vi "mydaq_equalizer.vi"() -> ()   [LabVIEW 2018]
uses:
  <vilib>/express/express analysis/Spectral/Block/exnSpectralBlock spectral measurements power poly.vi
  <vilib>/express/express analysis/Spectral/Block/exnSpectralBlock spectral measurements power DDT.vi
  <vilib>/express/express analysis/Spectral/XNode/ExpressSpectralMeasurementsBlockNode.xnode
panel:
  out "Waveform Graph":dynamicdata(graph)
  in  "Volume":dbl(slide) scale=0.0..1.0
  out "Slide 3":dbl(slide) scale=0.002..2.0
  out "Slide 2":dbl(slide) scale=0.002..2.0
  out "Slide":dbl(slide) scale=0.008..8.0
  in  "Bass":dbl(slide) scale=0.0..1.0
  in  "Midtone":dbl(slide) scale=0.0..1.0
  in  "Treble":dbl(slide)=0.5 scale=0.0..1.0
  in  "stop (F)":bool
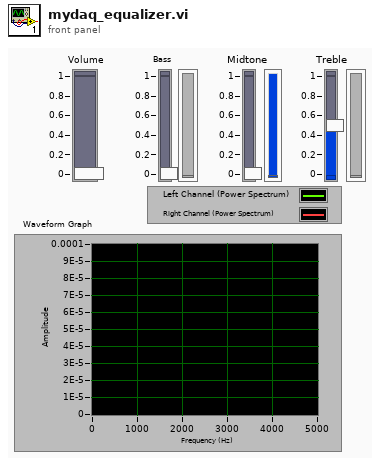
[diagram p1: front panel]
types:
  T1 = cluster{"averaging mode":u16, "weighting mode":u16, "number of averages":u32}
  T2 = cluster{"dB On (F)":bool, "unwrap phase (F)":bool, "convert to degree (F)":bool}
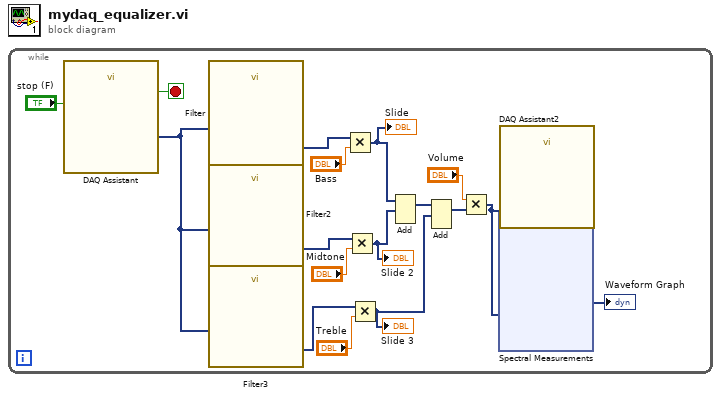
[diagram p0: block diagram]
diagram:
  n1 = while {
    stop <- w17 stop-if-true
    n2 = call "DAQ Assistant"("stop (F)"="stop (F)") -> ("data"=w15:dynamicdata, "stopped"=w17:bool)  [unwired: 15 in, 2 out]
    n3 = call "Filter"("Signal"=w15) -> ("Filtered Signal"=w11:dynamicdata)  [unwired: 9 in, 1 out]
    n4 = call "Filter2"("Signal"=w15) -> ("Filtered Signal"=w13:dynamicdata)  [unwired: 9 in, 1 out]
    n5 = call "Filter3"("Signal"=w15) -> ("Filtered Signal"=w9:dynamicdata)  [unwired: 9 in, 1 out]
    n6 = Multiply(x=w11, y="Bass") -> (x*y=w6:dynamicdata)
    "Slide" <- w6
    n7 = Multiply(x=w13, y="Midtone") -> (x*y=w5:dynamicdata)
    "Slide 2" <- w5
    n8 = Multiply(x=w9, y="Treble") -> (x*y=w7:dynamicdata)
    "Slide 3" <- w7
    n9 = Add(1:w5, 2:w6) -> (0:w14:dynamicdata)  [unwired: 1 in, 1 out]
    n10 = Add(1:w7, 2:w14) -> (0:w2:dynamicdata)  [unwired: 1 in, 1 out]
    n11 = Multiply(x="Volume", y=w2) -> (x*y=w4:dynamicdata)
    n12 = xnode "Spectral Measurements"("Signals"=w4) -> ("Power Spectrum"=→"Waveform Graph":dynamicdata)  [unwired: 1 in, 1 out]
    n13 = call "DAQ Assistant2"("data"=w4) -> ()  [unwired: 16 in, 3 out]
  }
